vi "Write Name.vi"(8 "error in (no error)":errorcluster, 10 "Name":string, 11 "IODevInfo in":refnum<class "IODevInfo.lvclass">) -> (0 "error out":errorcluster, 3 "IODevInfo out":refnum<class "IODevInfo.lvclass">)   [LabVIEW 2015, in "IODevInfo.lvclass"]
uses:
  IODevInfo.lvclass
  IODevInfo.lvclass/IODevInfo.ctl
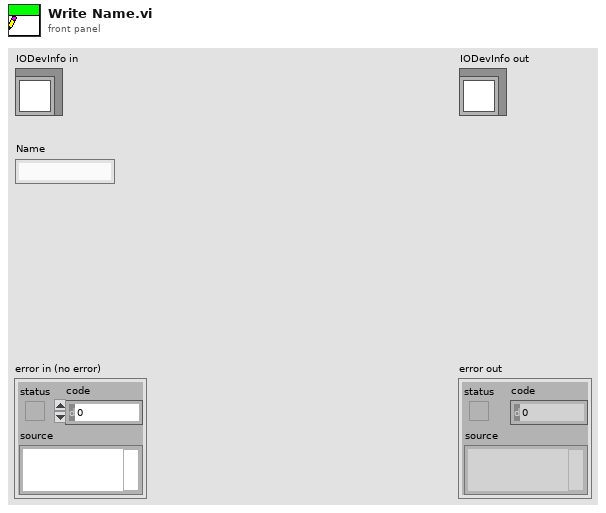
[diagram p1: front panel]
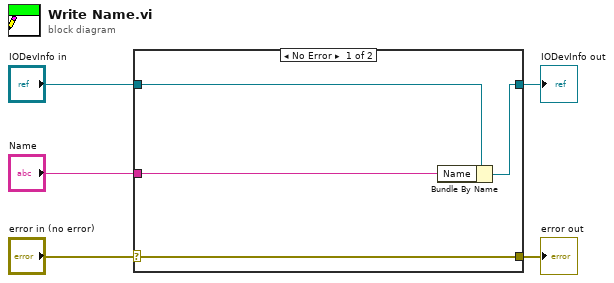
[diagram p0: block diagram]
diagram:
  n1 = case shown="No Error" "error in (no error)" {
    selector: "error in (no error)" -> [w9 w10]
    tunnel: [w9 w10] -> w4
    tunnel: [w7 w11] -> w2
    tunnel: "IODevInfo in" -> [w8 w11]
    tunnel: "Name" -> [w6 _]
    frame No Error {
      n2 = Bundle By Name(cluster=w8, "Name"=w6) -> (w7:refnum<class "IODevInfo.lvclass">)
    }
    frame Error {
    }
  }
  "error out" <- w4
  "IODevInfo out" <- w2
